vi "set_component_readiness.vi"(8 "error in (no error)":errorcluster, 9 "ready?":bool, 10 "top-level component type":T2=enum."ImagingMode", 11 "control references in":T1) -> (0 "error out":errorcluster, 3 "control references out":T1)   [LabVIEW 2010]
uses:
  type_definitions/clusters/controls_refs.ctl
  common/enumerations/top-level_component_type_enum.ctl
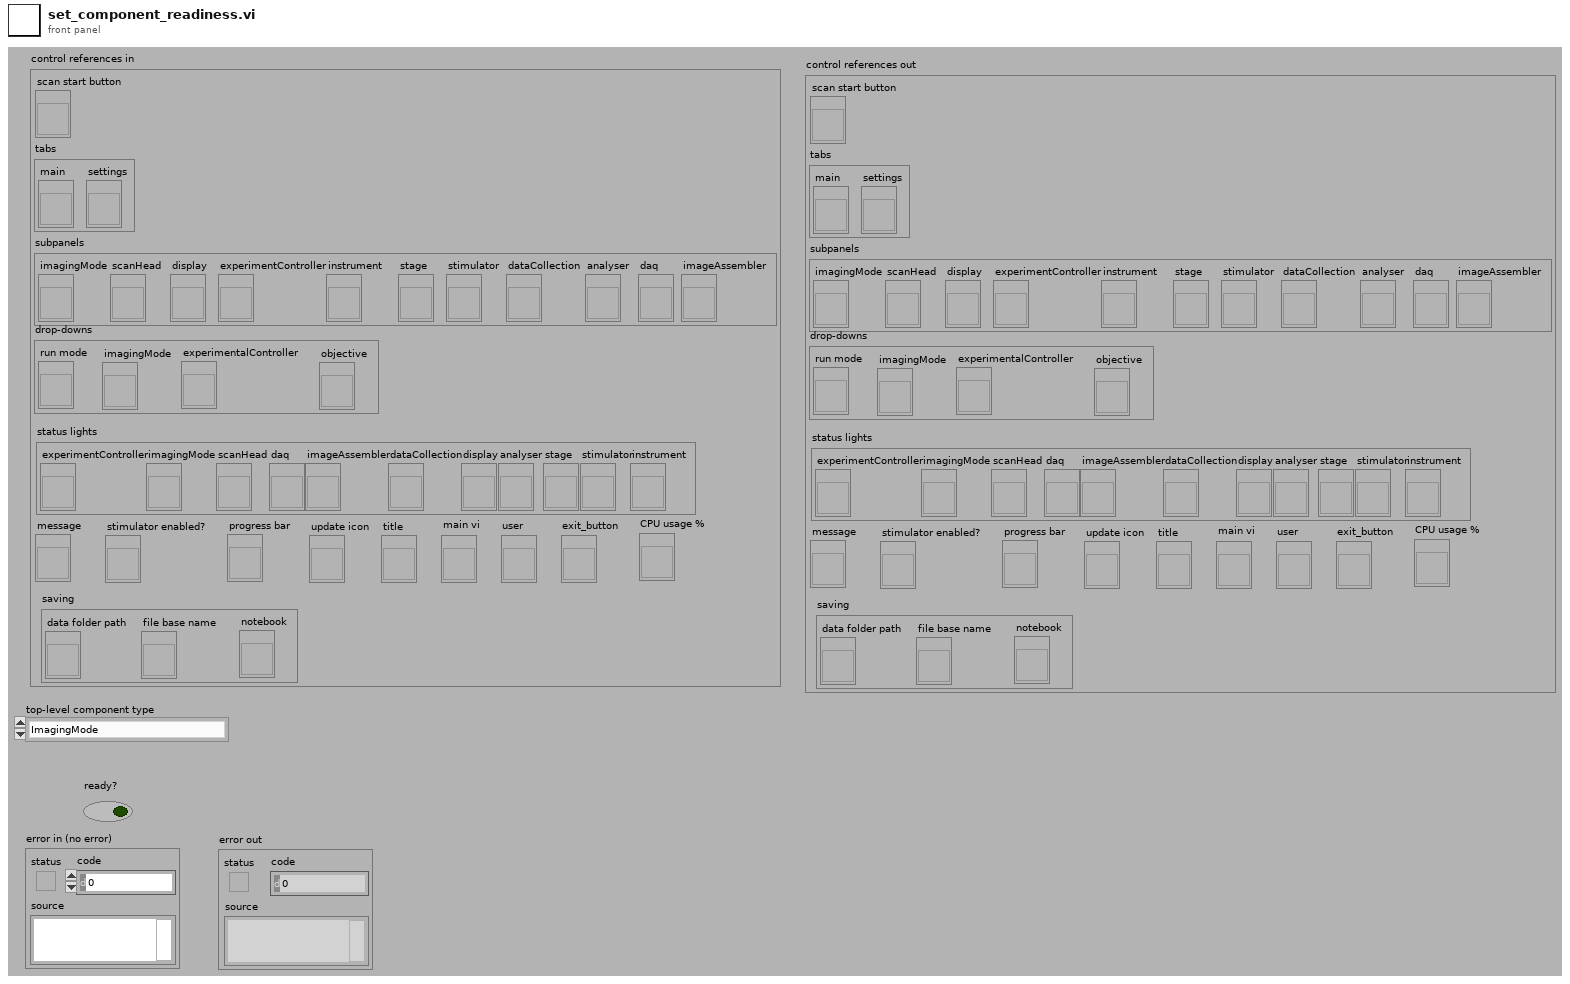
[diagram p1: front panel]
types:
  T1 = typedef "controls_refs.ctl" = cluster{"scan start button":refnum<vi>, "tabs":cluster{"main":refnum<vi>, "settings":refnum<vi>}, "subpanels":cluster{"imagingMode":refnum<vi>, "scanHead":refnum<vi>, "display":refnum<vi>, "experimentController":refnum<vi>, "instrument":refnum<vi>, "stage":refnum<vi>, "stimulator":refnum<vi>, "dataCollection":refnum<vi>, "analyser":refnum<vi>, "daq":refnum<vi>, "imageAssembler":refnum<vi>}, "drop-downs":cluster{"run mode":refnum<vi>, "imagingMode":refnum<vi>, "experimentalController":refnum<vi>, "objective":refnum<vi>}, "status lights":cluster{"experimentController":refnum<vi>, "imagingMode":refnum<vi>, "scanHead":refnum<vi>, "daq":refnum<vi>, "imageAssembler":refnum<vi>, "dataCollection":refnum<vi>, "display":refnum<vi>, "analyser":refnum<vi>, "stage":refnum<vi>, "stimulator":refnum<vi>, "instrument":refnum<vi>}, "message":refnum<vi>, "stimulator enabled?":refnum<vi>, "saving":cluster{"data folder path":refnum<vi>, "file base name":refnum<vi>, "notebook":refnum<vi>}, "progress bar":refnum<vi>, "update icon":refnum<vi>, "title":refnum<vi>, "main vi":refnum<vi>, "user":refnum<vi>, "exit_button":refnum<vi>, "CPU usage %":refnum<vi>}
  T2 = typedef "top-level_component_type_enum.ctl" = enum16{"undefined", "ImagingMode", "ScanHead", "DAQ", "ImageAssembler", "Display", "DataCollection", "Analyser", "Stimulator", "ExperimentController", "Instrument", "Stage"}
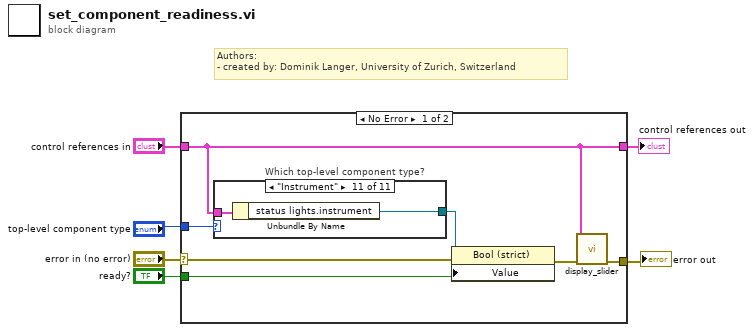
[diagram p0: block diagram]
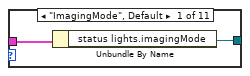
[diagram p2: hidden frame]
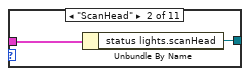
[diagram p3: hidden frame]
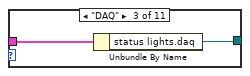
[diagram p4: hidden frame]
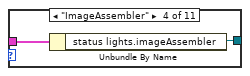
[diagram p5: hidden frame]
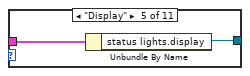
[diagram p6: hidden frame]
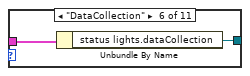
[diagram p7: hidden frame]
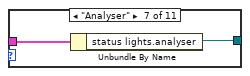
[diagram p8: hidden frame]
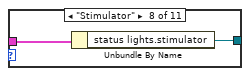
[diagram p9: hidden frame]
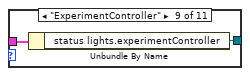
[diagram p10: hidden frame]
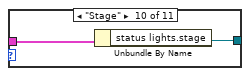
[diagram p11: hidden frame]
diagram:
  # "Authors: \n- created by: Dominik Langer, University of Zurich, Switzerland"
  n1 = case shown="No Error" "error in (no error)" {
    selector: "error in (no error)" -> [w12 w37]
    tunnel: "control references in" -> [w7 w36]
    tunnel: "ready?" -> [w11 _]
    tunnel: [w10 w37] -> w3
    tunnel: "top-level component type" -> [w8 _]
    tunnel: [w7 w36] -> w1
    frame No Error {
      n2 = case "Which top-level component type?" shown="\"Instrument\"" w8 {
        tunnel: w7 -> [w15 w17 w19 w21 w23 w25 w27 w29 w31 w32 w35]
        tunnel: [w14 w16 w18 w20 w22 w24 w26 w28 w30 w33 w34] -> w9
        frame "ImagingMode", Default {
          n3 = Unbundle By Name(w15) -> ("status lights.imagingMode"=w14:refnum<vi>)
        }
        frame "ScanHead" {
          n4 = Unbundle By Name(w17) -> ("status lights.scanHead"=w16:refnum<vi>)
        }
        frame "DAQ" {
          n5 = Unbundle By Name(w19) -> ("status lights.daq"=w18:refnum<vi>)
        }
        frame "ImageAssembler" {
          n6 = Unbundle By Name(w21) -> ("status lights.imageAssembler"=w20:refnum<vi>)
        }
        frame "Display" {
          n7 = Unbundle By Name(w23) -> ("status lights.display"=w22:refnum<vi>)
        }
        frame "DataCollection" {
          n8 = Unbundle By Name(w25) -> ("status lights.dataCollection"=w24:refnum<vi>)
        }
        frame "Analyser" {
          n9 = Unbundle By Name(w27) -> ("status lights.analyser"=w26:refnum<vi>)
        }
        frame "Stimulator" {
          n10 = Unbundle By Name(w29) -> ("status lights.stimulator"=w28:refnum<vi>)
        }
        frame "ExperimentController" {
          n11 = Unbundle By Name(w31) -> ("status lights.experimentController"=w30:refnum<vi>)
        }
        frame "Stage" {
          n12 = Unbundle By Name(w32) -> ("status lights.stage"=w33:refnum<vi>)
        }
        frame "Instrument" {
          n13 = Unbundle By Name(w35) -> ("status lights.instrument"=w34:refnum<vi>)
        }
      }
      n14 = property class="Bool (strict)"(reference=w9, error in=w12, "Value"=w11) -> (error out=w13:errorcluster)  [unwired: 1 out]
      n15 = call "display_slider.vi"("error in"=w13, "cluster refs in"=w7) -> ("error out"=w10:errorcluster)  [unwired: 9 in]
    }
    frame Error {
    }
  }
  "error out" <- w3
  "control references out" <- w1
